vi "AssertSubpanelVI.vi"(0 "VI Reference In":refnum<vi>, 1 "Label":string, 2 "delimiter (>>)":string=">>", 3 "Assert Only? (F)":bool, 5 "Control Path":string, 7 "VI Name":string, 11 "Error In":errorcluster, 12 "Assert Interval(10 ms)":u32=10, 13 "Timeout(5 sec)":dbl=5.0) -> (4 "VI Reference Out":refnum<vi>, 15 "Error Out":errorcluster)   [LabVIEW 2016, in "Drona.lvlib" / "AssertSubpanel.lvlib"]
doc: "Asserts the state of controls.\n\nThe input control name is given as a string , incase of path, use delimiters inbetween the path."
uses:
  AssertSubpanel.lvlib
  Get/GetControlRef/GetControlRefByPath.vi
  <vilib>/addons/_JKI Toolkits/Caraya/classes/Assert/Assert Equal Value_Variant.vi
  <vilib>/addons/_JKI Toolkits/Caraya/classes/Assert/Assert.lvclass
  Get/GetControlRef/GetControlRef.lvlib
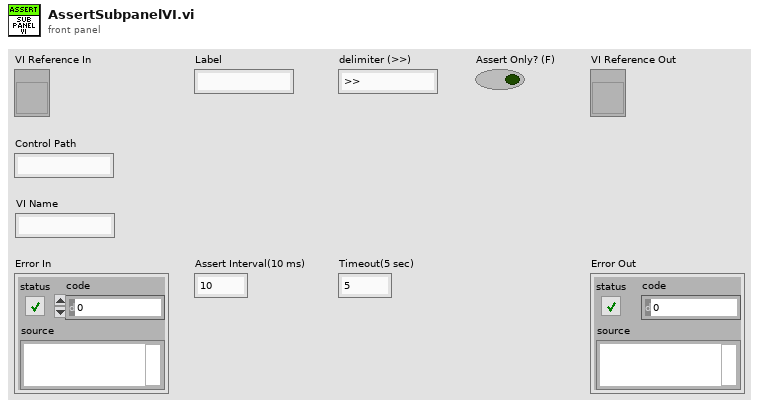
[diagram p1: front panel]
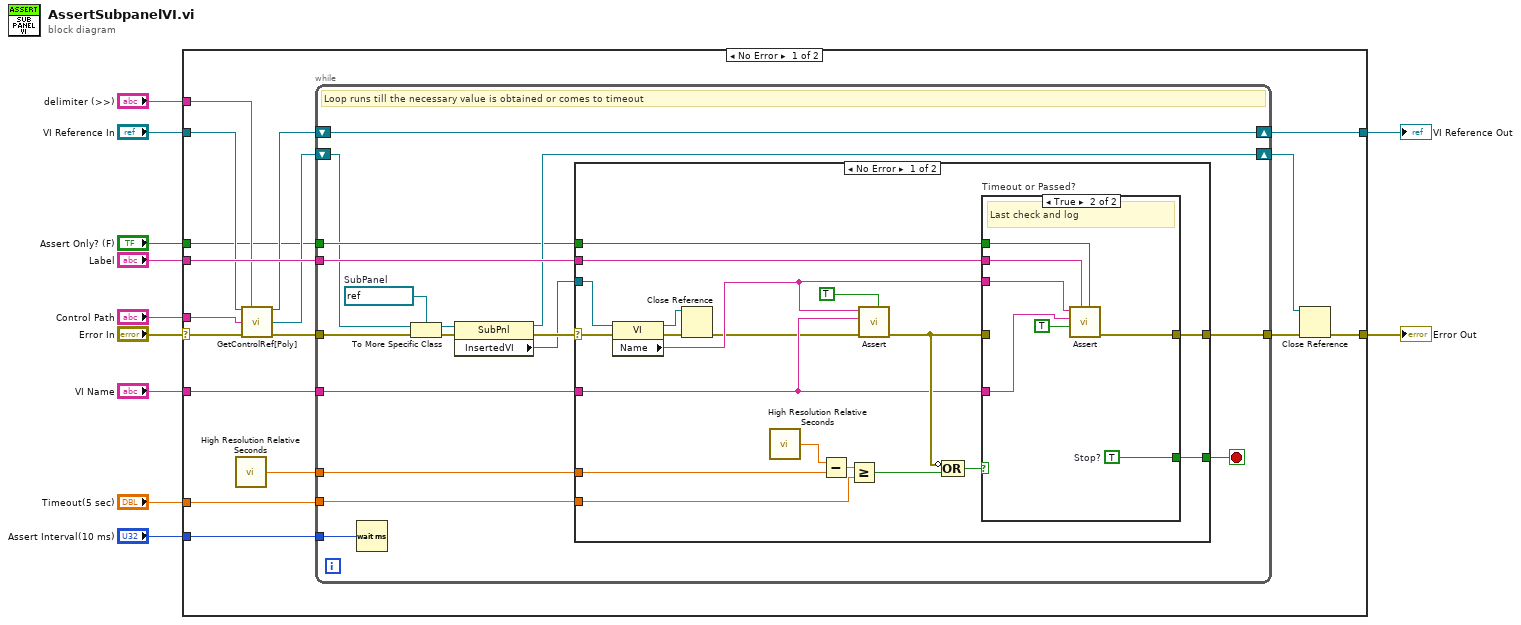
[diagram p0: block diagram]
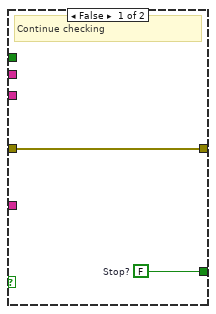
[diagram p2: hidden frame]
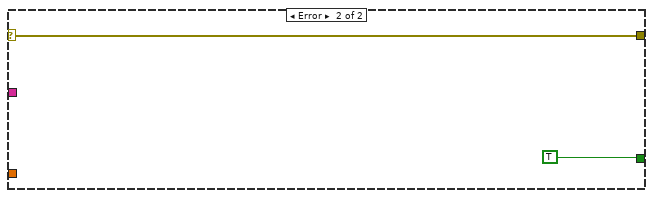
[diagram p3: hidden frame]
diagram:
  n1 = case shown="No Error" "Error In" {
    selector: "Error In" -> [w23 w77]
    tunnel: "Timeout(5 sec)" -> [w28 _]
    tunnel: [w27 w76] -> w10
    tunnel: [w16 w77] -> w9
    tunnel: "Assert Interval(10 ms)" -> [w25 _]
    tunnel: "Label" -> [w24 _]
    tunnel: "VI Reference In" -> [w22 w76]
    tunnel: "Control Path" -> [w21 _]
    tunnel: "delimiter (>>)" -> [w14 _]
    tunnel: "Assert Only? (F)" -> [w13 _]
    tunnel: "VI Name" -> [w12 _]
    frame No Error {
      n2 = call <vilib>:"High Resolution Relative Seconds.vi"() -> ("relative seconds"=w20:dbl)
      n3 = call-poly "GetControlRef[Poly].vi"("VI Reference In"=w22, "delimiter (>>)"=w14, "Control Path"=w21, "error In"=w23) -> ("VI Reference Out"=w18:refnum<vi>, "Ctl Refnum"=w17:refnum<vi>, "error out"=w19:errorcluster)  [unwired: 9 in]
      n4 = while {
        tunnel: w28 -> [w44]
        tunnel: w20 -> [w45]
        tunnel: w19 -> [w39]
        tunnel: [w42] -> w26
        tunnel: w25 -> [w40]
        tunnel: w24 -> [w37]
        shift-right: [w38] -> w27
        shift-left: w18 -> [w38]
        shift-right: [w36] -> w15
        shift-left: w17 -> [w30]
        tunnel: w13 -> [w35]
        tunnel: w12 -> [w33]
        stop <- w43 stop-if-true
        w31 = refnum<vi> refnum  # SubPanel
        # "Loop runs till the necessary value is obtained or comes to timeout"
        n5 = Wait (ms)(milliseconds to wait=w40) -> ()  [unwired: 1 out]
        n6 = To More Specific Class(target class=w31, reference=w30, error in=w39) -> (specific class reference=w29:refnum<vi>, error out=w32:errorcluster)
        n7 = property class="SubPnl"(reference=w29, error in=w32) -> (reference out=w36:refnum<vi>, error out=w41:errorcluster, "InsertedVI"=w34:refnum<vi>)
        n8 = case shown="No Error" w41 {
          selector: w41 -> [w49 w75]
          tunnel: w45 -> [w64 _]
          tunnel: w44 -> [w61 _]
          tunnel: [w54 TRUE] -> w43
          tunnel: [w55 w75] -> w42
          tunnel: w34 -> [w51 _]
          tunnel: w37 -> [w60 _]
          tunnel: w35 -> [w53 _]
          tunnel: w33 -> [w52 _]
          frame No Error {
            n9 = property class="VI"(reference=w51, error in=w49) -> (reference out=w46:refnum<vi>, error out=w48:errorcluster, "Name"=w50:string)
            n10 = Close Reference(reference=w46, error in (no error)=w48) -> (error out=w47:errorcluster)
            n11 = call <vilib>:"High Resolution Relative Seconds.vi"() -> ("relative seconds"=w63:dbl)
            n12 = Subtract(x=w63, y=w64) -> (x-y=w62:dbl)
            n13 = Greater Or Equal?(x=w62, y=w61) -> (x >= y?=w59:bool)
            n14 = call-poly <vilib>:"Assert.vi"("Assert Only? (F)"=TRUE, "error in (no error)"=w47, "Y"=w52, "X"=w50) -> ("error out"=w58:errorcluster)  [unwired: 7 in]
            n15 = Compound Arithmetic op=OR(invert w58, w59) -> (w57:bool)
            n16 = case "Timeout or Passed?" shown="True" w57 {
              tunnel: w58 -> [w66 _]
              tunnel: w50 -> [_ w72]
              tunnel: w60 -> [_ w73]
              tunnel: [w66 w71] -> w55
              tunnel: [w65 w70] -> w54
              tunnel: w53 -> [_ w68]
              tunnel: w52 -> [_ w67]
              frame False {
                w65 = FALSE  # Stop?
                # "Continue checking"
              }
              frame True {
                w70 = TRUE  # Stop?
                # "Last check and log"
                n17 = call-poly <vilib>:"Assert.vi"("Assert Only? (F)"=w68, "Label"=w73, "Register with caller test (F)"=TRUE, "Y"=w67, "X"=w72) -> ("error out"=w71:errorcluster)  [unwired: 6 in]
              }
            }
          }
          frame Error {
          }
        }
      }
      n18 = Close Reference(reference=w15, error in (no error)=w26) -> (error out=w16:errorcluster)
    }
    frame Error {
    }
  }
  "Error Out" <- w9
  "VI Reference Out" <- w10
